vi "aal_Complex Modulator(real input) (No State).vi"(6 "reset ?":bool, 7 "initial phase":dbl, 9 "fs":dbl=1024.0 min=-0.5 max=0.5 format="%.2f", 10 "frequency":dbl min=-0.5 max=0.5 format="%.2f", 11 "x":dbl[](array[numeric])) -> (3 "y":cdb[](array[numeric]), 5 "next initial phase":dbl)   [LabVIEW 2020, in "NI_AALPro.lvlib"]
doc: "Modulates the signal to frequency. The center frequency should be normalized (-0.5, 0.5)."
uses:
  <vilib>/Analysis/NI_AALPro.lvlib
  <resource>/lvanlys.dll
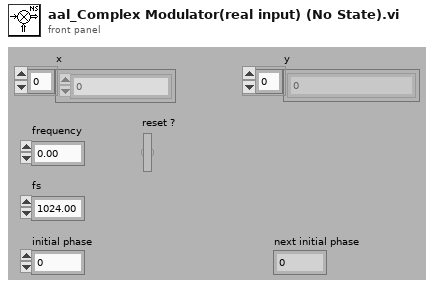
[diagram p1: front panel]
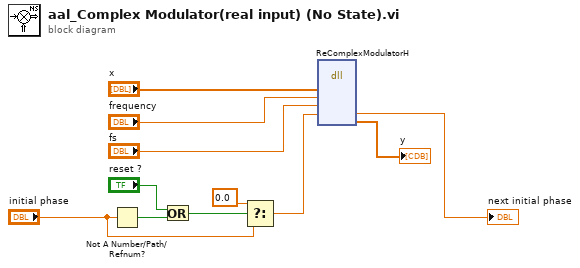
[diagram p0: block diagram]
diagram:
  n1 = Not A Number/Path/Refnum?(number/path/refnum="initial phase") -> (NaN/Path/Refnum?=w9:bool)
  n2 = Or(x="reset ?", y=w9) -> (x .or. y?=w4:bool)
  n3 = Select(t=0.0, s=w4, f="initial phase") -> (s? t:f=w5:dbl)
  n4 = dll-call lib="e:/builds/penguin/labview/branches/2020/dev/dist/resource/lvanlys.*" fn="ReComplexModulatorH"("xH"="x", "fc"="frequency", "fs"="fs", "initial_phase"=w5) -> ("initial_phase"=→"next initial phase":dbl, "y"=→"y":cdb[])  [unwired: 8 in, 2 out]
